vi "StatusParser.vi"(11 "Input String":string) -> (1 "Infusion rate(ul/s)":dbl, 2 "Infused Volume (ul)":dbl, 3 "Status":T1)   [LabVIEW 2020]
uses:
  Status_typeDef.ctl
  HarvardApp_PHDUltra_Pump.lvclass
panel:
  out "Array of Outputs":string[](array[string])
  out "Removed Motion Indicator":string
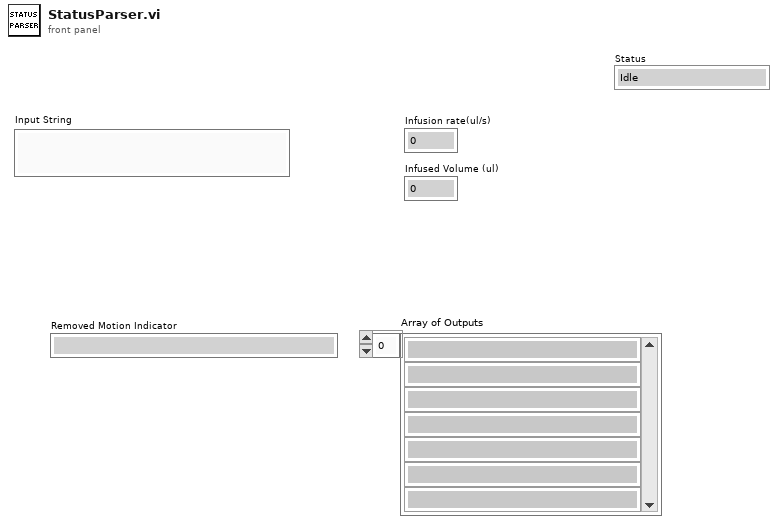
[diagram p1: front panel]
types:
  T1 = typedef "HarvardApp_PHDUltra_Pump.lvclass/Status_typeDef.ctl" = enum16{"Idle", "Infuse", "Moving", "Stalled", "Complete"}
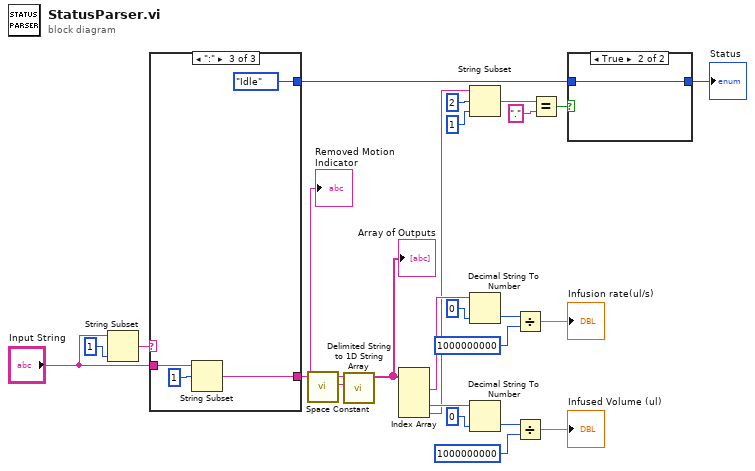
[diagram p0: block diagram]
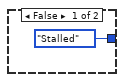
[diagram p2: hidden frame]
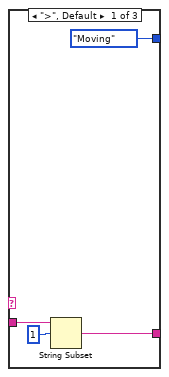
[diagram p3: hidden frame]
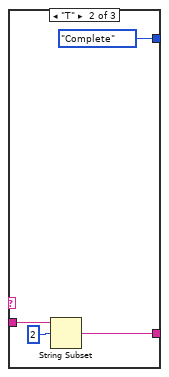
[diagram p4: hidden frame]
diagram:
  n1 = String Subset(string="Input String", length (rest)=1 ("length (rest)")) -> (substring=w23:string)  [unwired: 1 in]
  n2 = case shown="\":\"" w23 {
    tunnel: [Status_typeDef."Moving" ("Status") Status_typeDef."Complete" ("Status") Status_typeDef."Idle" ("Status")] -> w2
    tunnel: [w27 w31 w35] -> w21
    tunnel: "Input String" -> [w28 w30 w34]
    frame ">", Default {
      n3 = String Subset(string=w28, offset (0)=1) -> (substring=w27:string)  [unwired: 1 in]
    }
    frame "T" {
      n4 = String Subset(string=w30, offset (0)=2) -> (substring=w31:string)  [unwired: 1 in]
    }
    frame ":" {
      n5 = String Subset(string=w34, offset (0)=1) -> (substring=w35:string)  [unwired: 1 in]
    }
  }
  "Removed Motion Indicator" <- w21
  n6 = call "Space Constant.vi"() -> ("String"=w20:string)
  n7 = call "Delimited String to 1D String Array.vi"("delimiter"=w20, "delimited string"=w21) -> ("string array"=w19:string[])  [unwired: 9 in]
  "Array of Outputs" <- w19
  n8 = Index Array(array=w19) -> (element #1=w18:string, element #3=w9:string, element #4=w7:string)  [unwired: 4 in, 1 out]
  n9 = String Subset(string=w7, offset (0)=2, length (rest)=1 ("length (rest)")) -> (substring=w5:string)
  n10 = Decimal String To Number(string=w18, default (0L)=i64 0) -> (number=w16:i64)  [unwired: 1 in, 1 out]
  n11 = Decimal String To Number(string=w9, default (0L)=i64 0) -> (number=w11:i64)  [unwired: 1 in, 1 out]
  n12 = Divide(x=w16, y=i64 1000000000) -> (x/y=→"Infusion rate(ul/s)":dbl)
  n13 = Divide(x=w11, y=i64 1000000000) -> (x/y=→"Infused Volume (ul)":dbl)
  n14 = Equal?(x=w5, y=".") -> (x = y?=w3:bool)
  n15 = case shown="True" w3 {
    tunnel: w2 -> [_ w38]
    tunnel: [Status_typeDef."Stalled" ("Status") w38] -> w1
    frame False {
    }
    frame True {
    }
  }
  "Status" <- w1
